vi "Druck von Filterkammer ablassen.vi"(6 "Zustand":T2, 10 "DO 0-31":T1) -> (2 "DO 0-31":T1)   [LabVIEW 2020, in "Allgemein.lvlib"]
uses:
  Allgemein.lvlib
  Funktionstasten/Zustaende.ctl
  Verwaltung/Digital Ausgaenge 0-31.ctl
  Funktionstasten/Funktionstasten.lvlib
  Verwaltung/Verwaltung - cRIO.lvlib
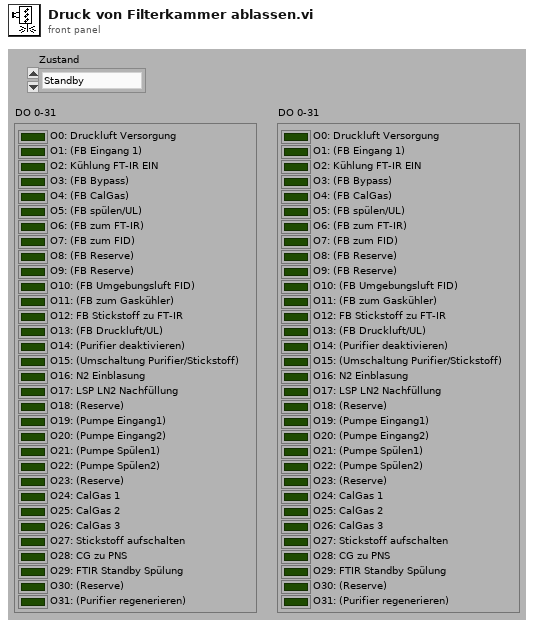
[diagram p1: front panel]
types:
  T1 = typedef "Verwaltung - cRIO.lvlib/Digital Ausgaenge 0-31.ctl" = cluster{"O0: Druckluft Versorgung":bool, "O1: (FB Eingang 1)":bool, "O2: Kühlung FT-IR EIN":bool, "O3: (FB Bypass)":bool, "O4: (FB CalGas)":bool, "O5: (FB spülen/UL)":bool, "O6: (FB zum FT-IR)":bool, "O7: (FB zum FID)":bool, "O8: (FB Reserve)":bool, "O9: (FB Reserve)":bool, "O10: (FB Umgebungsluft FID)":bool, "O11: (FB zum Gaskühler)":bool, "O12: FB Stickstoff zu FT-IR":bool, "O13: (FB Druckluft/UL)":bool, "O14: (Purifier deaktivieren)":bool, "O15: (Umschaltung Purifier/Stickstoff)":bool, "O16: N2 Einblasung":bool, "O17: LSP LN2 Nachfüllung":bool, "O18: (Reserve)":bool, "O19: (Pumpe Eingang1)":bool, "O20: (Pumpe Eingang2)":bool, "O21: (Pumpe Spülen1)":bool, "O22: (Pumpe Spülen2)":bool, "O23: (Reserve)":bool, "O24: CalGas 1":bool, "O25: CalGas 2":bool, "O26: CalGas 3":bool, "O27: Stickstoff aufschalten":bool, "O28: CG zu PNS":bool, "O29: FTIR Standby Spülung":bool, "O30: (Reserve)":bool, "O31: (Purifier regenerieren)":bool}
  T2 = typedef "Funktionstasten.lvlib/Zustaende.ctl" = enum16{"Standby", "Pause", "Eco", "Messen", "Kalibrieren", "Spülen Filter", "Spülen Leitung", "Umgebungsluft", "0-Gas", "Cal-Gas", "CG zu PNS", "-------------", "Init 1", "Init 2", "Init 3", "Init 4", "Messen vorbereiten", "Messen durchführen", "Exit"}
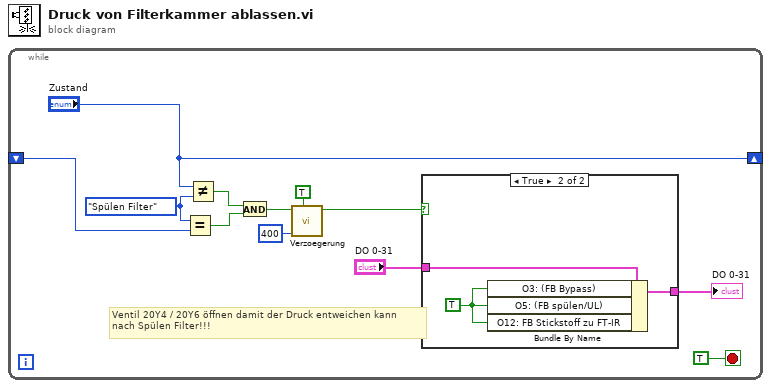
[diagram p0: block diagram]
diagram:
  n1 = while {
    shift-right: ["Zustand"] -> _
    shift-left: _ -> [w5]
    stop <- TRUE stop-if-true
    w11 = Zustaende."Spülen Filter" ("y")
    # "Ventil 20Y4 / 20Y6 öffnen damit der Druck entweichen kann\nnach Spülen Filter!!!"
    n2 = Equal?(x=w11, y=w5) -> (x = y?=w9:bool)
    n3 = Not Equal?(x="Zustand", y=w11) -> (x != y?=w10:bool)
    n4 = And(x=w10, y=w9) -> (x .and. y?=w8:bool)
    n5 = call "Verzoegerung.vi"("Abfallverzögerung?"=TRUE, "ms"=u16 400, "Startsignal"=w8) -> ("Zeit abgelaufen?"=w1:bool)  [unwired: 7 in, 1 out]
    n6 = case shown="True" w1 {
      tunnel: "DO 0-31" -> [w13 w16]
      tunnel: [w13 w15] -> w2
      frame False {
      }
      frame True {
        w14 = TRUE ("O3: FB Bypass")
        n7 = Bundle By Name(cluster=w16, "O3: (FB Bypass)"=w14, "O5: (FB spülen/UL)"=w14, "O12: FB Stickstoff zu FT-IR"=w14) -> (w15:T1)
      }
    }
    "DO 0-31" <- w2
  }
